vi "Application Name--constant.vi"() -> (3 "Application Name":string="Rename As Application Name")   [LabVIEW 2020, in "Rename as Application Shared.lvlib"]
uses:
  Rename as Application Shared.lvlib
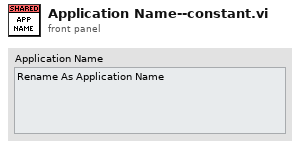
[diagram p1: front panel]
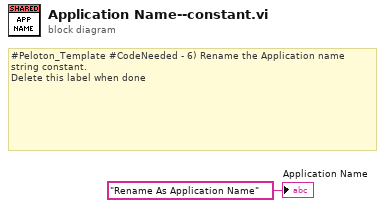
[diagram p0: block diagram]
diagram:
  # "#Peloton_Template #CodeNeeded - 6) Rename the Application name string constant.\nDelete this label when done"
  "Application Name" <- "Rename As Application Name"
